vi "string history.vi"(10 "State Queue":string) -> (2 "State Queue history (last on top)":string)   [LabVIEW 2019]
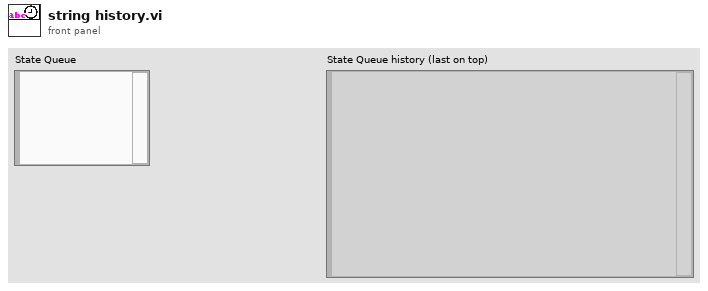
[diagram p1: front panel]
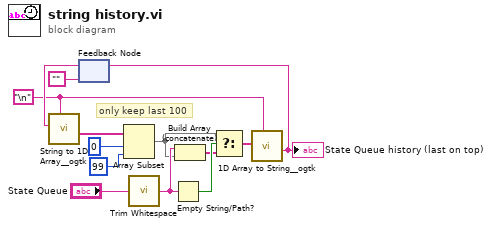
[diagram p0: block diagram]
diagram:
  w6 = "\n"
  # "only keep last 100"
  n1 = feedback #1("" ("delimited string")) -> (w9:string)
  n2 = call <userlib>:"String to 1D Array__ogtk.vi"("delimiter (Tab)"=w6, "string"=w9) -> ("Array of Strings"=w13:string[])  [unwired: 9 in]
  n3 = Array Subset(array=w13, index=0 ("length"), length=99 ("index")) -> (w1:string[])
  n4 = call <vilib>:"Trim Whitespace.vi"("string"="State Queue") -> ("trimmed string"=w5:string)  [unwired: 1 in]
  n5 = Empty String/Path?(string/path=w5) -> (empty?=w4:bool)
  n6 = Build Array (concatenate)(w5, w1) -> (w3:string[])
  n7 = Select(t=w1, s=w4, f=w3) -> (s? t:f=w2:string[])
  n8 = call <userlib>:"1D Array to String__ogtk.vi"("delimiter (Tab)"=w6, "Array of Strings"=w2) -> ("delimited string"=w10:string)  [unwired: 9 in]
  "State Queue history (last on top)" <- w10
  n9 = feedback-in #1(w10) -> ()
